vi "setSampling.vi"(8 "error in (no error)":errorcluster, 10 "sampling":T1={"Fs"=204789.0, "#s"=15753}, 11 "Instrument.LockinAPI in":refnum<class "Instrument.LockinAPI.lvclass">) -> (0 "error out":errorcluster, 3 "Instrument.LockinAPI out":refnum<class "Instrument.LockinAPI.lvclass">)   [LabVIEW 2019, in "Instrument.LockinAPI.lvclass"]
doc: "API to put lockin into remote mode.\n\nIf address=\"\", this API reads from localhost\nIf address is remote lockin, you need to add this computer to allowed whitelist on the lockin computer you are trying to access."
uses:
  Instrument.LockinAPI.lvclass
  Typedefs/API/LockinAPI.Sampling.Sampling--Cluster.ctl
  C:/Users/patrick/Documents/GitHub/Instrument-Framework/lvsrc/Instrument/Instrument.lvclass
  Typedefs/API/LockinAPI.Commands--Enum.ctl
  Typedefs/API/LockinAPI.Sampling.FsMode--enum.ctl
  3bf1471f-c9f6-40c5-b66e-4f6cc53cda49.vi
  3bf1471f-c9f6-40c5-b66e-4f6cc53cda49.vi/a5837a2d-f7fb-4e40-a24d-e1b13ec832b6.vi
  3bf1471f-c9f6-40c5-b66e-4f6cc53cda49.vi/a5837a2d-f7fb-4e40-a24d-e1b13ec832b6.vi/03197671-f2a3-4037-a8bc-432b0a4227a5.vi
  3bf1471f-c9f6-40c5-b66e-4f6cc53cda49.vi/a5837a2d-f7fb-4e40-a24d-e1b13ec832b6.vi/db7b4c25-5cae-45ee-b867-46adefe1772c.vi
  3bf1471f-c9f6-40c5-b66e-4f6cc53cda49.vi/a5837a2d-f7fb-4e40-a24d-e1b13ec832b6.vi/f7a3782b-2d62-4130-8e43-22cad49b27e6.vi
  <vilib>/JDP Science/JSONtext/Make JSON Array.vi
  3bf1471f-c9f6-40c5-b66e-4f6cc53cda49.vi/a5837a2d-f7fb-4e40-a24d-e1b13ec832b6.vi/db7b4c25-5cae-45ee-b867-46adefe1772c.vi/81697911-d5ff-4c7a-b88f-2b2862327f84.vi
  3bf1471f-c9f6-40c5-b66e-4f6cc53cda49.vi/a5837a2d-f7fb-4e40-a24d-e1b13ec832b6.vi/f7a3782b-2d62-4130-8e43-22cad49b27e6.vi/5a625396-7887-4cc1-855e-9786433f6466.vi
  3bf1471f-c9f6-40c5-b66e-4f6cc53cda49.vi/a5837a2d-f7fb-4e40-a24d-e1b13ec832b6.vi/f7a3782b-2d62-4130-8e43-22cad49b27e6.vi/fcbc9424-eb8a-451e-95eb-1680c01f3b08.vi
  Instrument/API/Enum to String.vi
  Instrument/Private/Get RC Connection Status.vi
  <vilib>/JDP Science/JSONtext/Variant to JSON Text.vi
  <vilib>/JDP Science/JSONtext/support/Format JSON Array Text.vi
  Instrument/API/Send and Receive.vi
  <vilib>/JDP Science/JSONtext/JSON text to Variant.vi
  <vilib>/Utility/Data Type/Get Type Information.vi
  <vilib>/JDP Science/JSONtext/LVClass Serializer/JSONtext LVClass Serializer.lvclass
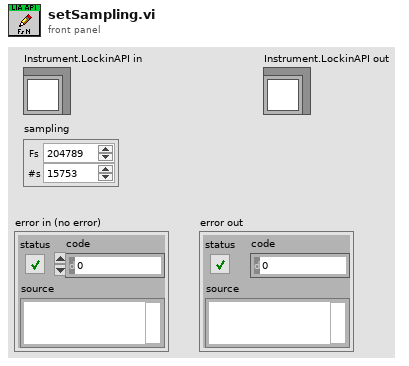
[diagram p1: front panel]
types:
  T1 = typedef "Instrument.LockinAPI.lvclass/LockinAPI.Sampling.Sampling--Cluster.ctl" = cluster{"Fs":dbl, "#s":i32}
  T2 = typedef "Instrument.LockinAPI.lvclass/LockinAPI.Sampling.FsMode--enum.ctl" = enum16{"Manual", "Auto Fs", "Max Fs"}
  T3 = typedef "Instrument.LockinAPI.lvclass/LockinAPI.Commands--Enum.ctl" = enum16{"setAI", "setAO", "setAO_Amplitude", "setAO_DC", "setAO_Frequency", "setAO_Phase", "setAO_Function", "setAO_I+", "setREF", "setREF_Frequency", "setREF_Phase", "setREF_TC", "setREF_Roll-Off", "setDAQ", "setSampling", "setOffset", "setState", "getState", "getAO", "getAI", "getResults", "getSampling", "getAOconfig", "getREFconfig", "setInputGain", "setOutputGain", "getInputGain", "getOutputGain", "setSamplingMode", "getSamplingMode", "setSweep", "setSweepTime", "setSweepTable", "getStatus", "getSweepResults", "getSweepWaveforms", "startSweep", "stopSweep", "setAUX", "getAUX"}
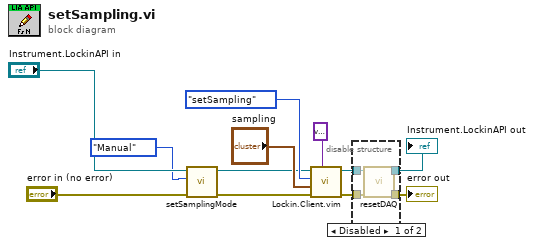
[diagram p0: block diagram]
diagram:
  n1 = call-dynamic "setSamplingMode.vi"("error in (no error)"="error in (no error)", "Fs Mode"=LockinAPI.Sampling.FsMode--enum."Manual", "Instrument.LockinAPI in"="Instrument.LockinAPI in") -> ("error out"=w8:errorcluster, "Instrument.LockinAPI out"=w7:refnum<class "Instrument.LockinAPI.lvclass">)  [unwired: 7 in]
  n2 = call "Lockin.Client.vim"("Data Out type"=variant, "error in (no error)"=w8, "Data"="sampling", "Command"=LockinAPI.Commands--Enum."setSampling", "Instrument.LockinAPI in"=w7) -> ("error out"=w3:errorcluster, "Instrument.LockinAPI out"=w6:refnum<class "Instrument.LockinAPI.lvclass">)  [unwired: 4 in, 1 out]
  n3 = disable-structure shown="Disabled" {
    disable-tunnel: w6 -> [w16 w18]
    disable-tunnel: [w15 w18] -> w5
    disable-tunnel: [w14 w17] -> w4
    disable-tunnel: w3 -> [w13 w17]
    frame Disabled {
      n4 = call "resetDAQ.vi"("error in (no error)"=w13, "Instrument.LockinAPI in"=w16) -> ("error out"=w14:errorcluster, "Instrument.LockinAPI out"=w15:refnum<class "Instrument.LockinAPI.lvclass">)  [unwired: 8 in]
    }
    frame Enabled {
    }
  }
  "error out" <- w4
  "Instrument.LockinAPI out" <- w5
